vi "test Export Custom Device.vi"(8 "error in (no error)":errorcluster, 11 "TestCase in":refnum<class "Routing and Faulting Export Unit Tests.lvclass">) -> (0 "error out":errorcluster, 3 "TestCase out":refnum<class "Routing and Faulting Export Unit Tests.lvclass">)   [LabVIEW 2020, in "Routing and Faulting Export Unit Tests.lvclass"]
uses:
  Routing and Faulting Export Unit Tests.lvclass
  <vilib>/NI/NI VeriStand Advanced SysDef API/_Types/TreeItem.ctl
  <vilib>/NI/NI VeriStand Advanced SysDef API/_Types/TreeItem.Info.ctl
  <vilib>/NI VeriStand/Custom Device API/Custom Device Channel.ctl
  <vilib>/NI VeriStand/Custom Device API/Custom Device Channel Type.ctl
  <vilib>/NI VeriStand/Custom Device API/Custom Device Waveform.ctl
  <vilib>/NI VeriStand/Custom Device API/Custom Device Waveform DataType.ctl
  <vilib>/NI/NI VeriStand Advanced SysDef API/_Types/TreeItem.Property.ctl
  Routing and Faulting Export Unit Tests.lvclass/Routing and Faulting Export Unit Tests.ctl
  <vilib>/addons/_JKI Toolkits/VI Tester/TestCase.llb/TestCase.lvclass
  <vilib>/NI/NI VeriStand Advanced SysDef API/SysDef API/Advanced System Definition.lvlib
  <vilib>/NI VeriStand/Custom Device API/Custom Device API.lvlib
  C:/Program Files (x86)/National Instruments/LabVIEW 2020/vi.lib/addons/_JKI Toolkits/VI Tester/TestCase.llb/TestCase.lvclass
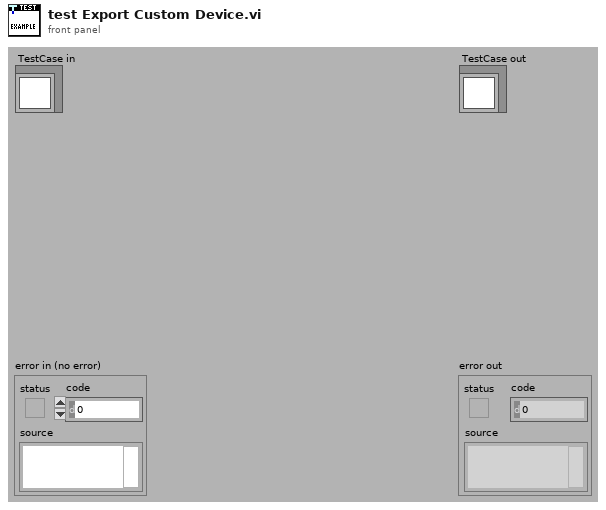
[diagram p1: front panel]
types:
  T1 = typedef "Advanced System Definition.lvlib/TreeItem.ctl" = cluster{"Item Info":T2, "Parent Path":string[], "Properties":T7[]}
  T2 = typedef "Advanced System Definition.lvlib/TreeItem.Info.ctl" = cluster{"Name":string, "Description":string, "GUID":string, "Is Channel":bool, "Channel":T3, "Is Waveform":bool, "Waveform":T5}
  T3 = typedef "Custom Device API.lvlib/Custom Device Channel.ctl" = cluster{"Type":T4, "Units":string, "Default Value":dbl, "Faultable":bool, "Scalable":bool}
  T4 = typedef "Custom Device API.lvlib/Custom Device Channel Type.ctl" = enum16{"Input", "Output"}
  T5 = typedef "Custom Device API.lvlib/Custom Device Waveform.ctl" = cluster{"Data Type":T6, "Units":string}
  T6 = typedef "Custom Device API.lvlib/Custom Device Waveform DataType.ctl" = enum16{"Double", "Complex Double"}
  T7 = typedef "Advanced System Definition.lvlib/TreeItem.Property.ctl" = cluster{"Name":string, "Type":i32, "Value":variant}
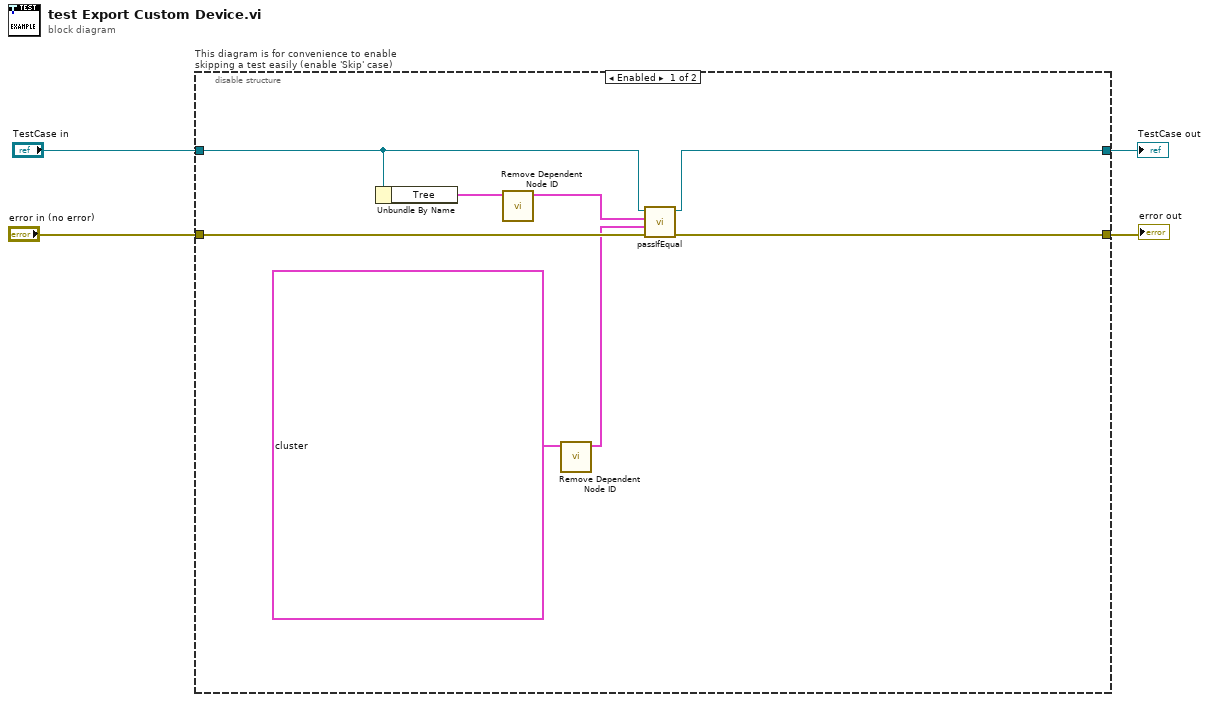
[diagram p0: block diagram]
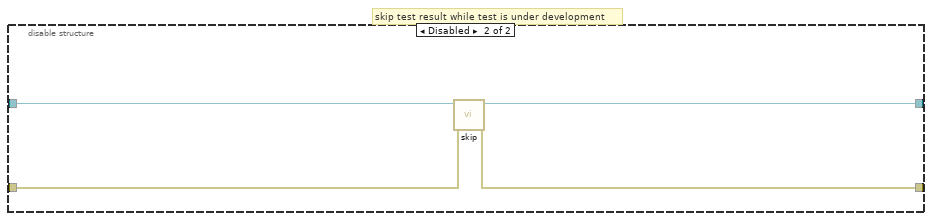
[diagram p2: hidden frame]
diagram:
  n1 = disable-structure "This diagram is for convenience to enable skipping a test easily (enable 'Skip' case)" shown="Enabled" {
    disable-tunnel: "TestCase in" -> [w11 w16]
    disable-tunnel: [w10 w14] -> w1
    disable-tunnel: [w9 w15] -> w3
    disable-tunnel: "error in (no error)" -> [w12 w13]
    frame Enabled {
      n2 = Unbundle By Name(w11) -> ("Tree"=w6:T1[])
      n3 = call "Remove Dependent Node ID.vi"("Tree In"=w6) -> ("Tree Out"=w8:T1[])  [unwired: 10 in]
      n4 = call "Remove Dependent Node ID.vi"("Tree In"=T1[] [{"Item Info"={"Name"="Routing and Faulting", "Description"="", "GUID"="4e591626-626d-4903-9a6e-1f2a7b879f4d", "Is Channel"=FALSE, "Channel"={"Type"=enum."Input", "Units"="", "Default Value"=0.0, "Faultable"=FALSE, "Scalable"=FALSE}, "Is Waveform"=FALSE, "Waveform"={"Data Type"=enum."Double", "Units"=""}}, "Parent Path"=["Targets", "Controller", "Custom Devices"], "Properties"=[{"Name"="user.CD.Modules", "Type"=14, "Value"=variant(string[] ["0", "1"])}, {"Name"="user.CD.Modules.0", "Type"=8, "Value"=variant(string "Hardware/SLSC/SLSC Chassis/Modules/Slot 2 (SLSC Switch)", "VS.ASD.TreeItem.DependentNodeID"=variant(u64 196), "VS.ASD.TreeItem.DependentNodeType"=variant(bool FALSE))}, {"Name"="user.CD.Modules.1", "Type"=8, "Value"=variant(string "Hardware/SLSC/SLSC Chassis/Modules/Slot 4 (SLSC Switch)", "VS.ASD.TreeItem.DependentNodeID"=variant(u64 202), "VS.ASD.TreeItem.DependentNodeType"=variant(bool FALSE))}]}, {"Item Info"={"Name"="Endpoint Aliases", "Description"="", "GUID"="58f3342d-82ee-4932-869a-6f49da3049e5", "Is Channel"=FALSE, "Channel"={"Type"=enum."Input", "Units"="", "Default Value"=0.0, "Faultable"=FALSE, "Scalable"=FALSE}, "Is Waveform"=FALSE, "Waveform"={"Data Type"=enum."Double", "Units"=""}}, "Parent Path"=["Targets", "Controller", "Custom Devices", "Routing and Faulting"], "Properties"=[{"Name"="user.CD.Slot 2 Alias 0", "Type"=0, "Value"=variant(string "0,DUT_Ch0", "IsBinary"=variant(bool FALSE))}, {"Name"="user.CD.Slot 2 Alias 1", "Type"=0, "Value"=variant(string "0,LOAD_Ch0", "IsBinary"=variant(bool FALSE))}, {"Name"="user.CD.Slot 4 Alias 0", "Type"=0, "Value"=variant(string "1,DUT_Ch0", "IsBinary"=variant(bool FALSE))}, {"Name"="user.CD.Slot 4 Alias 1", "Type"=0, "Value"=variant(string "1,LOAD_Ch0", "IsBinary"=variant(bool FALSE))}]}, {"Item Info"={"Name"="Routing Channels", "Description"="", "GUID"="ce8870b5-cb8e-4b52-ac34-5b792fdc2ead", "Is Channel"=FALSE, "Channel"={"Type"=enum."Input", "Units"="", "Default Value"=0.0, "Faultable"=FALSE, "Scalable"=FALSE}, "Is Waveform"=FALSE, "Waveform"={"Data Type"=enum."Double", "Units"=""}}, "Parent Path"=["Targets", "Controller", "Custom Devices", "Routing and Faulting"], "Properties"=[]}, {"Item Info"={"Name"="Empty Channel", "Description"="Empty Channel", "GUID"="7ecc8b72-3e89-41fd-aa1c-b993e8fe884f", "Is Channel"=TRUE, "Channel"={"Type"=enum."Input", "Units"="", "Default Value"=-1.0, "Faultable"=FALSE, "Scalable"=FALSE}, "Is Waveform"=FALSE, "Waveform"={"Data Type"=enum."Double", "Units"=""}}, "Parent Path"=["Targets", "Controller", "Custom Devices", "Routing and Faulting", "Routing Channels"], "Properties"=[{"Name"="Value Table", "Type"=15, "Value"=variant("No Connections"=variant(cluster{"index":i32, "key":string, "value":variant} {"index"=0, "key"="No Connections", "value"=variant(dbl -1.0)}), "VS.ASD.TreeItem.DictType"=variant(string "Double"))}, {"Name"="user.CD.Connections", "Type"=15, "Value"=variant("No Connections"=variant(cluster{"index":i32, "key":string, "value":variant} {"index"=0, "key"="No Connections", "value"=variant(string[] [])}), "VS.ASD.TreeItem.DictType"=variant(string "ArrayStringProperty"))}, {"Name"="user.CD.Descriptions", "Type"=15, "Value"=variant("No Connections"=variant(cluster{"index":i32, "key":string, "value":variant} {"index"=0, "key"="No Connections", "value"=variant(string "State with no connections")}), "VS.ASD.TreeItem.DictType"=variant(string "String"))}]}, {"Item Info"={"Name"="Routing Channel", "Description"="This channel has some trivial states in it.", "GUID"="7ecc8b72-3e89-41fd-aa1c-b993e8fe884f", "Is Channel"=TRUE, "Channel"={"Type"=enum."Input", "Units"="", "Default Value"=0.0, "Faultable"=FALSE, "Scalable"=FALSE}, "Is Waveform"=FALSE, "Waveform"={"Data Type"=enum."Double", "Units"=""}}, "Parent Path"=["Targets", "Controller", "Custom Devices", "Routing and Faulting", "Routing Channels"], "Properties"=[{"Name"="Value Table", "Type"=15, "Value"=variant("No Connections"=variant(cluster{"index":i32, "key":string, "value":variant} {"index"=0, "key"="No Connections", "value"=variant(dbl -1.0)}), "One Connection"=variant(cluster{"index":i32, "key":string, "value":variant} {"index"=1, "key"="One Connection", "value"=variant(dbl 0.0)}), "Two Connections"=variant(cluster{"index":i32, "key":string, "value":variant} {"index"=2, "key"="Two Connections", "value"=variant(dbl 10.0)}), "VS.ASD.TreeItem.DictType"=variant(string "Double"))}, {"Name"="user.CD.Connections", "Type"=15, "Value"=variant("No Connections"=variant(cluster{"index":i32, "key":string, "value":variant} {"index"=0, "key"="No Connections", "value"=variant(string[] [])}), "One Connection"=variant(cluster{"index":i32, "key":string, "value":variant} {"index"=1, "key"="One Connection", "value"=variant(string[] ["0,DUT_Ch0,LOAD_Ch0"])}), "Two Connections"=variant(cluster{"index":i32, "key":string, "value":variant} {"index"=2, "key"="Two Connections", "value"=variant(string[] ["1,DUT_Ch0,LOAD_Ch0", "0,DUT_Ch0,LOAD_Ch0"])}), "VS.ASD.TreeItem.DictType"=variant(string "ArrayStringProperty"))}, {"Name"="user.CD.Descriptions", "Type"=15, "Value"=variant("No Connections"=variant(cluster{"index":i32, "key":string, "value":variant} {"index"=0, "key"="No Connections", "value"=variant(string "State with no connections")}), "One Connection"=variant(cluster{"index":i32, "key":string, "value":variant} {"index"=1, "key"="One Connection", "value"=variant(string "One connection in this state")}), "Two Connections"=variant(cluster{"index":i32, "key":string, "value":variant} {"index"=2, "key"="Two Connections", "value"=variant(string "Two connections in this state")}), "VS.ASD.TreeItem.DictType"=variant(string "String"))}]}, {"Item Info"={"Name"="Status", "Description"="", "GUID"="fafe2633-52e8-4be6-bb95-b07e42834d60", "Is Channel"=FALSE, "Channel"={"Type"=enum."Input", "Units"="", "Default Value"=0.0, "Faultable"=FALSE, "Scalable"=FALSE}, "Is Waveform"=FALSE, "Waveform"={"Data Type"=enum."Double", "Units"=""}}, "Parent Path"=["Targets", "Controller", "Custom Devices", "Routing and Faulting"], "Properties"=[]}, {"Item Info"={"Name"="Heartbeat", "Description"="Running count used for debugging. If this channel continues to increment, the custom device is still executing.", "GUID"="03D3BB99-1485-13A6-561D1F898F032919", "Is Channel"=TRUE, "Channel"={"Type"=enum."Output", "Units"="", "Default Value"=0.0, "Faultable"=FALSE, "Scalable"=FALSE}, "Is Waveform"=FALSE, "Waveform"={"Data Type"=enum."Double", "Units"=""}}, "Parent Path"=["Targets", "Controller", "Custom Devices", "Routing and Faulting", "Status"], "Properties"=[]}, {"Item Info"={"Name"="Status Code", "Description"="Status code of the custom device. A negative value indicates failure. A positive value indicates warning.", "GUID"="03D3BB99-1485-13A6-561D1F898F032919", "Is Channel"=TRUE, "Channel"={"Type"=enum."Output", "Units"="", "Default Value"=0.0, "Faultable"=FALSE, "Scalable"=FALSE}, "Is Waveform"=FALSE, "Waveform"={"Data Type"=enum."Double", "Units"=""}}, "Parent Path"=["Targets", "Controller", "Custom Devices", "Routing and Faulting", "Status"], "Properties"=[]}] ("Export.Tree")) -> ("Tree Out"=w7:T1[])  [unwired: 10 in]
      n5 = call-dynamic "passIfEqual.vi"("error in (no error)"=w12, "y"=w7, "x"=w8, "TestCase in"=w11) -> ("error out"=w9:errorcluster, "TestCase out"=w10:refnum<class "Routing and Faulting Export Unit Tests.lvclass">)  [unwired: 6 in]
    }
    frame Disabled {
      # "skip test result while test is under development"
      n6 = call <vilib>:"skip.vi"("error in (no error)"=w13, "TestCase in"=w16) -> ("error out"=w15:errorcluster, "TestCase out"=w14:refnum<class "Routing and Faulting Export Unit Tests.lvclass">)  [unwired: 8 in]
    }
  }
  "error out" <- w3
  "TestCase out" <- w1
